vi "validate configuration.vi"(8 "error in":errorcluster, 11 "configuration in":refnum<class "TBM module configuration.lvclass">) -> (0 "error out":errorcluster, 3 "configuration out":refnum<class "TBM module configuration.lvclass">)   [LabVIEW 2013, in "TBM module configuration.lvclass"]
doc: "Provides an interface for performing validation on a given configuration. Any children should define the behavior of this function to ensure that the configuration in memory can be used by the runtime class."
uses:
  TBM module configuration.lvclass
  root configuration/TBM configuration.lvclass
  <vilib>/NI/Tag Bus/tag/tag descriptor.lvclass/tag descriptor.ctl
  <vilib>/NI/Tag Bus/tag/read tag name.vi
  <vilib>/NI/Tag Bus/tag/read data type.vi
  channel/TBM channel.lvclass
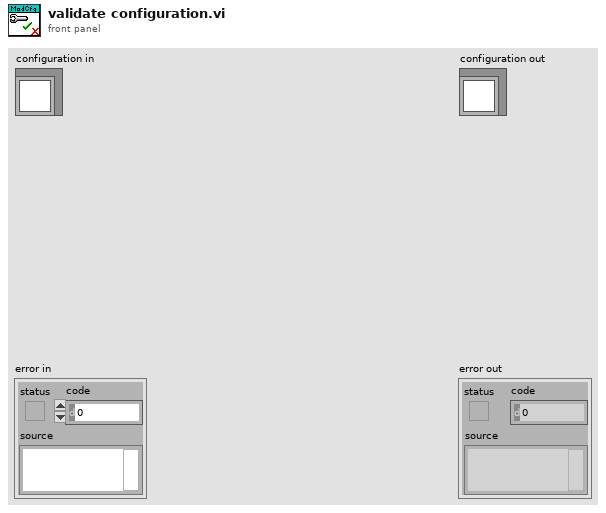
[diagram p1: front panel]
types:
  T1 = typedef "tag bus.lvlib/tag descriptor.lvclass/Data Type.ctl" = enum16{"Double", "Single", "I64", "I32", "I16", "I8", "U64", "U32", "U16", "U8", "Boolean", "String", "Array of Double", "Array of Single", "Array of I64", "Array of I32", "Array of I16", "Array of I8", "Array of U64", "Array of U32", "Array of U16", "Array of U8", "Array of Boolean", "Array of String"}
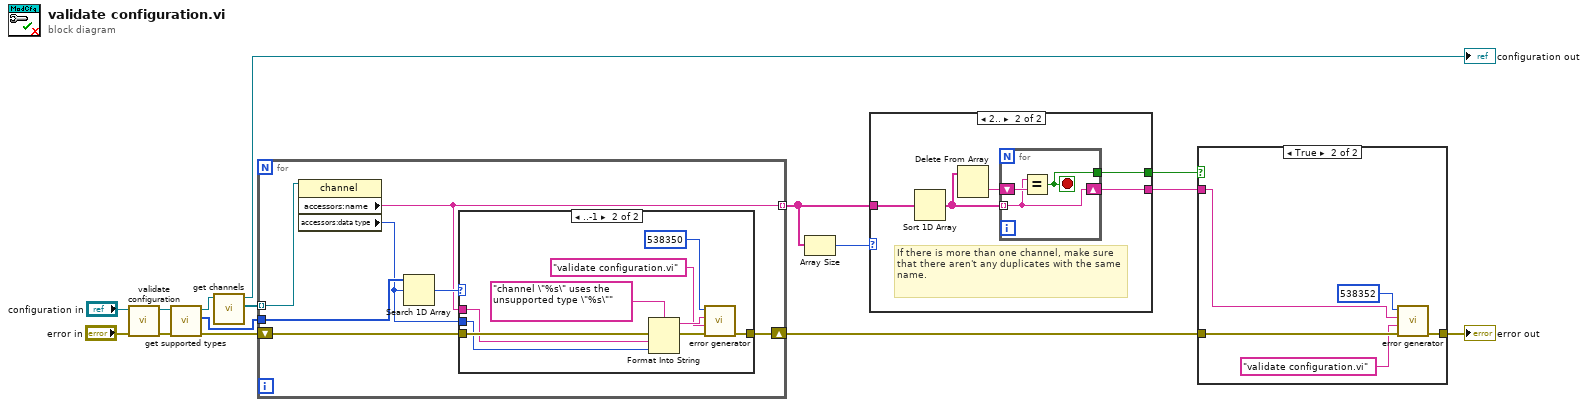
[diagram p0: block diagram]
diagram:
  n1 = call-parent "validate configuration.vi"("error in"="error in", "configuration in"="configuration in") -> ("error out"=w13:errorcluster, "configuration out"=w12:refnum<class "TBM module configuration.lvclass">)  [unwired: 8 in]
  n2 = call-dynamic "get supported types.vi"("error in"=w13, "module configuration in"=w12) -> ("error out"=w8:errorcluster, "supported types"=w9:T1[], "module configuration out"=w11:refnum<class "TBM module configuration.lvclass">)  [unwired: 7 in]
  n3 = call-dynamic "get channels.vi"("module configuration in"=w11) -> ("channels"=w10:refnum<class "TBM channel.lvclass">[], "module configuration out"=→"configuration out":refnum<class "TBM module configuration.lvclass">)  [unwired: 9 in]
  n4 = for {
    tunnel: w10 -> [w22] mode=indexing
    tunnel: w9 -> [w21]
    shift-right: [w18] -> w5
    shift-left: w8 -> [w19]
    tunnel: [w16] -> w2 mode=indexing
    n5 = property class="channel"(reference=w22) -> ("accessors:name"=w16:string, "accessors:data type"=w17:T1)  [unwired: 1 in, 2 out]
    n6 = Search 1D Array(1D array=w21, element=w17) -> (index of element=w20:i32)  [unwired: 1 in]
    n7 = case shown="..-1" w20 {
      tunnel: w19 -> [w23 w27]
      tunnel: [w23 w26] -> w18
      tunnel: w17 -> [_ w25]
      tunnel: w16 -> [_ w24]
      frame 0.. {
      }
      frame ..-1 {
        n8 = Format Into String(format string="channel \"%s\" uses the unsupported type \"%s\"", error in=w27, w24, w25) -> (resulting string=w30:string, error out=w31:errorcluster)  [unwired: 1 in]
        n9 = call "error generator.vi"("error in"=w31, "source"="validate configuration.vi" ("format string"), "append error message"=w30, "error code (0)"=538350) -> ("error out"=w26:errorcluster)  [unwired: 7 in]
      }
    }
  }
  n10 = Array Size(array=w2) -> (size(s)=w1:i32)
  n11 = case shown="2.." w1 {
    tunnel: [_ w35] -> w4
    tunnel: [_ w34] -> w3
    tunnel: w2 -> [_ w33]
    frame ..1 {
    }
    frame 2.. {
      # "If there is more than one channel, make sure that there aren't any duplicates with the same name."
      n12 = Sort 1D Array(array=w33) -> (sorted array=w36:string[])
      n13 = Delete From Array(array=w36) -> (deleted portion=w37:string)  [unwired: 2 in, 1 out]
      n14 = for {
        shift-right: [w39] -> w34
        shift-left: w37 -> [w40]
        tunnel: w36 -> [w39] mode=indexing
        tunnel: [w38] -> w35
        stop <- w38 stop-if-true
        n15 = Equal?(x=w39, y=w40) -> (x = y?=w38:bool)
      }
    }
  }
  n16 = case shown="True" w4 {
    tunnel: w5 -> [w41 w45]
    tunnel: [w41 w46] -> w6
    tunnel: w3 -> [_ w44]
    frame False {
    }
    frame True {
      n17 = call "error generator.vi"("error in"=w45, "source"="validate configuration.vi" ("format string"), "append error message"=w44, "error code (0)"=538352) -> ("error out"=w46:errorcluster)  [unwired: 7 in]
    }
  }
  "error out" <- w6
